vi "Config File View.vi"(0 "Path":path, 2 "File View":bool, 13 "Channel 1":T2(array[cluster]) {"Stop Bit" items=["1.0", "1.5", "2.0"]; "Parity" items=["None", "Odd", "Even", "Mark", "Space"]}, 14 "OK Button":bool) -> (17 "concatenated string":string, 19 "data":T1(array[cluster]))   [LabVIEW 2020]
panel:
  in  "Cancel Button":bool
  in  "Text Ring":u16(ring)
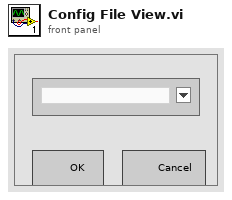
[diagram p1: front panel]
types:
  T1 = cluster{"Port No.":refnum<visa-resource-name>, "Checkbox":bool, "Parity":u16, "Stop Bit":u16, "Baud Rate":dbl, "Data Bits":dbl}[]
  T2 = cluster{"Port No.":refnum<visa-resource-name>, "Checkbox":bool, "Parity":u16, "Stop Bit":u16, "Baud Rate":u32, "Data Bits":u8}[]
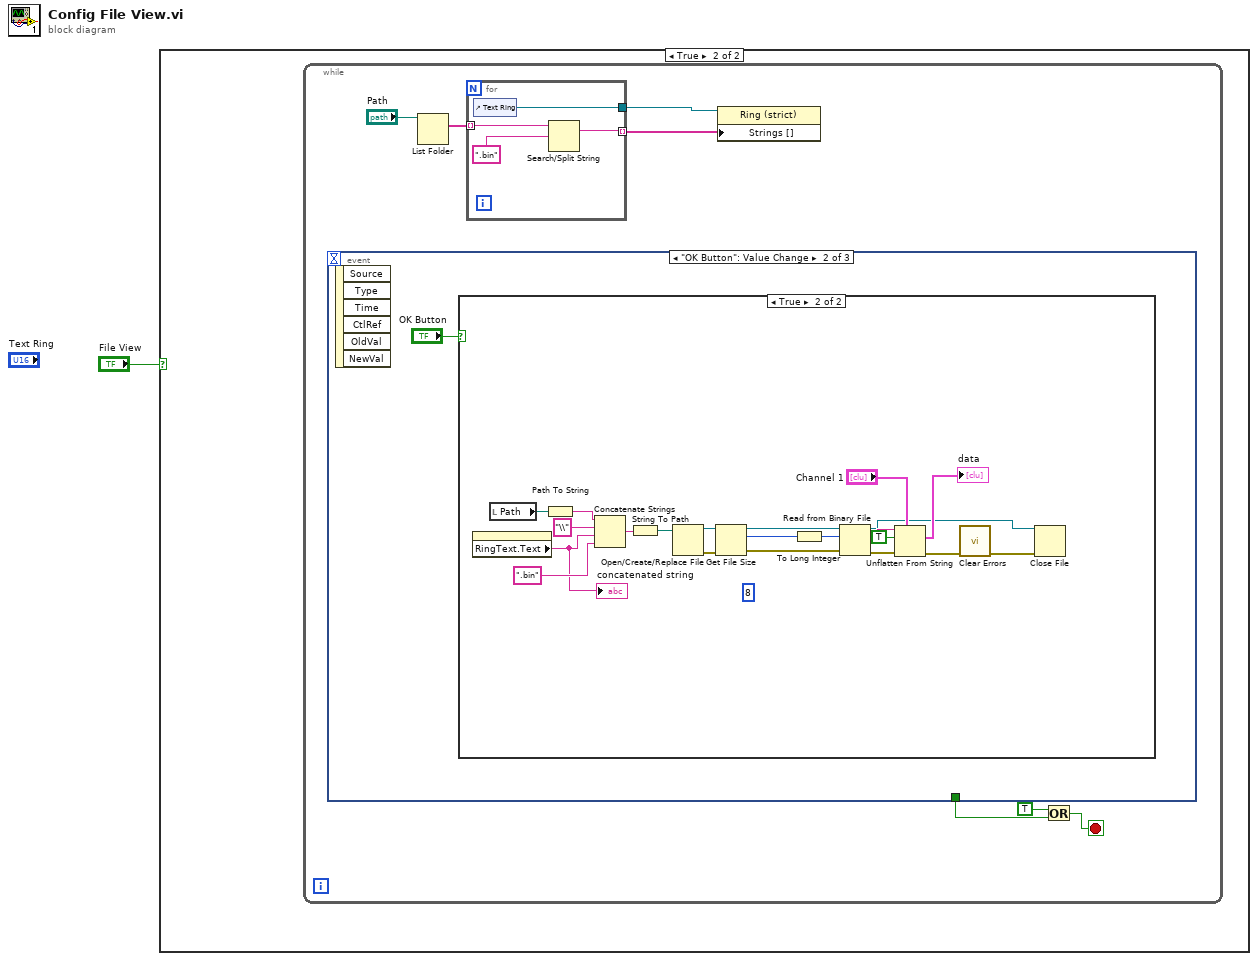
[diagram p0: block diagram]
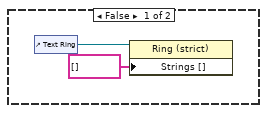
[diagram p2: hidden frame]
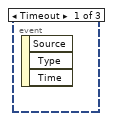
[diagram p3: hidden frame]
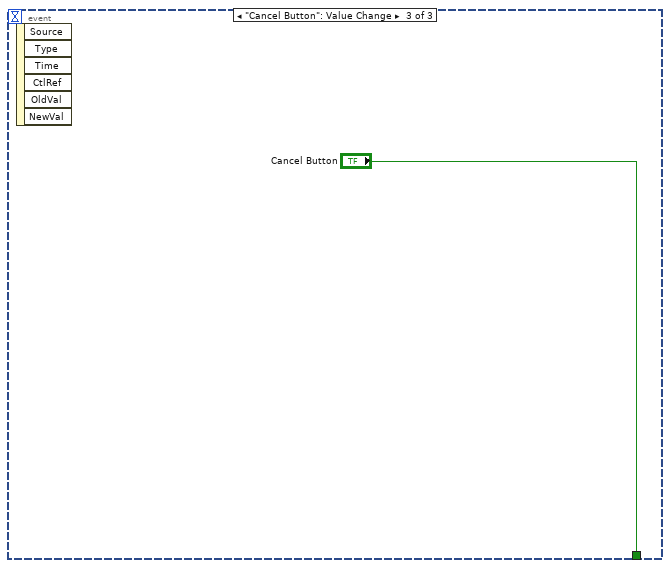
[diagram p5: hidden frame]
diagram:
  n1 = case shown="True" "File View" {
    frame False {
      n2 = control-ref of="Text Ring"() -> (w3:refnum<vi>)
      n3 = property on="Property Node" class="Ring (strict)"(reference=w3, "Strings []"=string[] []) -> ()  [unwired: 1 in, 2 out]
    }
    frame True {
      n4 = while {
        stop <- w9 stop-if-true
        n5 = event shown="[1] \"OK Button\": Value Change" {
          selector: _ -> [_ _ _]
          dyn-events: _ -> [_ _ _]
          timeout: _ -> [_ _ _]
          tunnel: [_ _ "Cancel Button"] -> w6
          event Timeout {
            n6 = event-data() -> ()  [unwired: 1 in, 3 out]
          }
          event "OK Button": Value Change {
            n7 = event-data() -> ()  [unwired: 1 in, 6 out]
            n8 = case shown="True" "OK Button" {
              frame False {
              }
              frame True {
                (unwired) i64 8 ("y")
                n9 = property on="Text Ring" class="Ring (strict)"() -> ("RingText.Text"=w29:string)  [unwired: 2 in, 2 out]
                "concatenated string" <- w29
                n10 = local read "Path"() -> (w36:path)
                n11 = Path To String(path=w36) -> (string=w35:string)
                n12 = Concatenate Strings(w35, "\\" ("string"), w29, ".bin" ("string")) -> (w33:string)
                n13 = String To Path(string=w33) -> (path=w32:path)
                n14 = Open/Create/Replace File(file path (use dialog)=w32) -> (refnum out=w26:refnum<file>, error out=w31:errorcluster)  [unwired: 5 in, 1 out]
                n15 = Get File Size(file=w26, error in=w31) -> (refnum out=w28:refnum<file>, size (in bytes)=w17:i64, 0:w27:errorcluster)
                n16 = To Long Integer(number=w17) -> (32bit integer=w16:i32)
                n17 = Read from Binary File(8:w27, 10:w16, 11:w28) -> (0:w23:errorcluster, 2:w24:string, 3:w18:refnum<file>)  [unwired: 3 in, 1 out]
                n18 = Unflatten From String(type="Channel 1", binary string=w24, data includes array or string size? (T)=TRUE, error in (no error)=w23) -> (value=→"data":T2, error out=w22:errorcluster)  [unwired: 1 in, 1 out]
                n19 = call <vilib>:"Clear Errors.vi"("error in (no error)"=w22) -> ("error out"=w25:errorcluster)  [unwired: 5 in, 1 out]
                n20 = Close File(refnum=w18, error in=w25) -> ()  [unwired: 2 out]
              }
            }
          }
          event "Cancel Button": Value Change {
            n21 = event-data() -> ()  [unwired: 1 in, 6 out]
          }
        }
        n22 = List Folder(path="Path") -> (filenames=w8:string[])  [unwired: 3 in, 3 out]
        n23 = for {
          tunnel: w8 -> [w14] mode=indexing
          tunnel: [w12] -> w5
          tunnel: [w11] -> w4 mode=indexing
          n24 = control-ref of="Text Ring"() -> (w12:refnum<vi>)
          n25 = Search/Split String(string=w14, search string/char (-)=".bin") -> (substring before match=w11:string)  [unwired: 1 in, 2 out]
        }
        n26 = property on="Property Node" class="Ring (strict)"(reference=w5, "Strings []"=w4) -> ()  [unwired: 1 in, 2 out]
        n27 = Or(x=TRUE, y=w6) -> (x .or. y?=w9:bool)
      }
    }
  }
